vi "grabarVideoSinGuardar.vi"(0 "VideoMode":u32=20, 3 "Quality":u32=500, 5 "Stop (F)":bool, 7 "error in":errorcluster, 8 "Image Logging Path":string="C:\\Users\\TGM1603\\Documents\\Videos", 9 "Frame Rate":u32=30) -> (20 "Image Out":T1(plugin-control), 26 "Stopped":bool, 27 "error out":errorcluster)   [LabVIEW 2024]
doc: "Creates, and edits acquisitions using the NI Vision Acquisition Express VI.\n\nThe NI Vision Acquisition Wizard is launched by placing the Express VI on the block diagram. Select an acquisition source and configure an acquisition using NI-IMAQ, NI-IMAQdx, or simulate an acquisition by reading an AVI or image files from a folder. After an acquisition is configured, select controls and indicators to be able to programmatically set in LabVIEW. Double-click the Vision Acquisition Express VI to edit the acquisition.\n\nNote: Any images created by the Express VI need to be disposed after use. Use the IMAQ Dispose.vi to cleanup the images output by the Express VI when they are no longer needed."
uses:
  <vilib>/vision/driver/Vision Acquisition Express Utility VIs.llb/Vision Acquisition Path Convert (String).vi
  <vilib>/vision/driver/NI_Vision_Acquisition_Software.lvlib
  <resource>/objmgr/imaqdx.rc
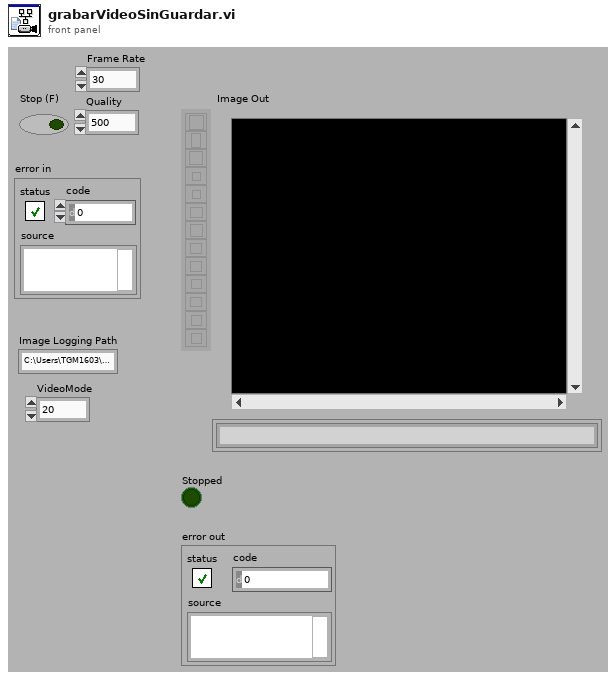
[diagram p1: front panel]
types:
  T1 = typedef "IMAQ Image.ctl" = refnum<image>
  T2 = typedef "IMAQdx.ctl" = refnum<k21>
  T3 = cluster{"File Type":string, "Quality":u32, "Compress":bool, "Lossless":bool, "Ratio":sgl, "Codec":string, "Frame Rate":u32, "Limit Frames":bool, "Max Frames":u32}
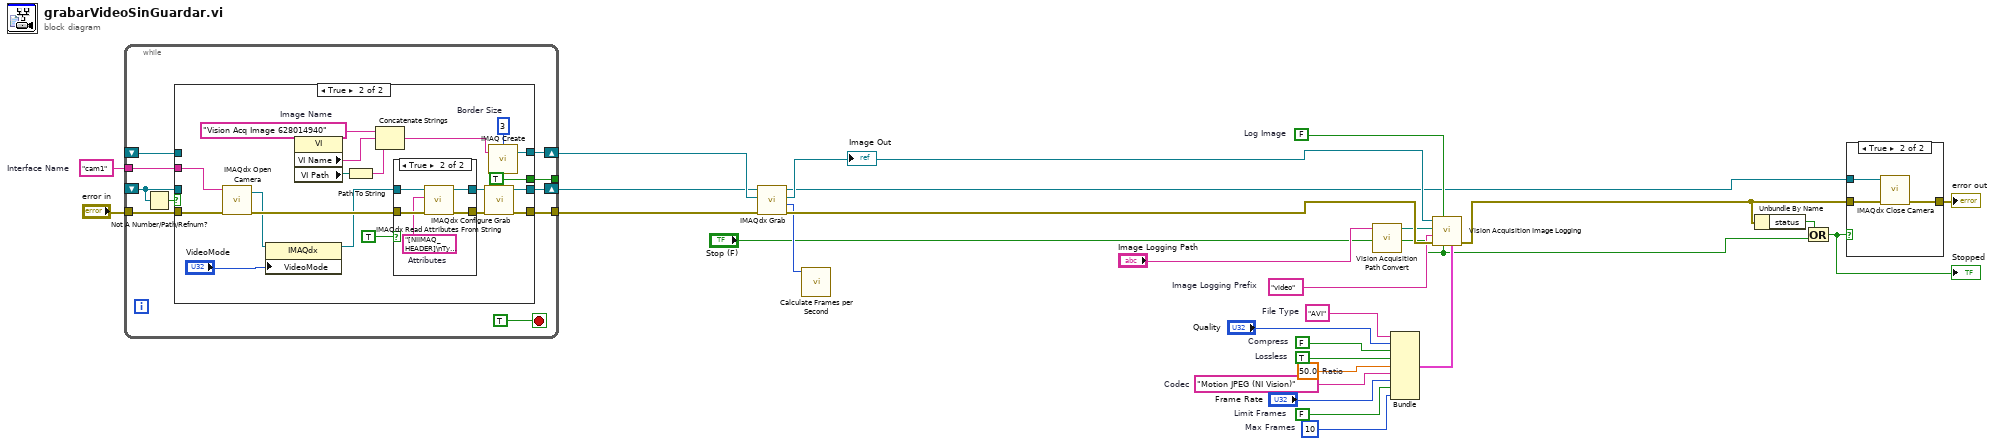
[diagram p0: block diagram]
diagram:
  w9 = FALSE  # Log Image
  w20 = "video"  # Image Logging Prefix
  w15 = sgl 50.0  # Ratio
  w16 = TRUE  # Lossless
  w17 = FALSE  # Compress
  w14 = "Motion JPEG (NI Vision)"  # Codec
  w11 = u32 10  # Max Frames
  w12 = FALSE  # Limit Frames
  w19 = "AVI"  # File Type
  w26 = "cam1"  # Interface Name
  n1 = while "While Loop_template0" {
    shift-right: [w38] -> w24
    shift-left: _ -> [w31]
    tunnel: [w37] -> w27
    tunnel: "error in" -> [w36]
    shift-right: [w34] -> w25
    shift-left: _ -> [w33]
    tunnel: w26 -> [w32]
    tunnel: [w29] -> _
    stop <- TRUE ("_template0") stop-if-true
    n2 = Not A Number/Path/Refnum?(number/path/refnum=w31) -> (NaN/Path/Refnum?=w30:bool)
    n3 = case "Case Structure_template0" shown="True" w30 {
      tunnel: [w41 w59] -> w38
      tunnel: w31 -> [w41 _]
      tunnel: [w40 w58] -> w37
      tunnel: w36 -> [w40 w60]
      tunnel: [w39 w57] -> w34
      tunnel: w33 -> [w39 _]
      tunnel: w32 -> [_ w48]
      tunnel: [_ TRUE] -> w29
      frame False {
      }
      frame True {
        w45 = 3  # Border Size
        w52 = "Vision Acq Image 628014940"  # Image Name
        n4 = call <vilib>:"IMAQdx Open Camera.vi"("error in"=w60, "Session In"=w48) -> ("error out"=w51:errorcluster, "Session Out"=w43:T2)  [unwired: 1 in, 7 out]
        n5 = property class="IMAQdx"(reference=w43, "VideoMode"="VideoMode") -> (reference out=w42:T2)  [unwired: 1 in, 1 out]
        n6 = property class="VI"() -> ("VI Name"=w55:string, "VI Path"=w56:path)  [unwired: 2 in, 2 out]
        n7 = Path To String(path=w56) -> (string=w54:string)
        n8 = Concatenate Strings(w52, w55, w54) -> (w53:string)
        n9 = case shown="True" TRUE ("Init Attributes") {
          tunnel: w42 -> [w62 w67]
          tunnel: w51 -> [w61 w66]
          tunnel: [w62 w64] -> w50
          tunnel: [w61 w63] -> w49
          frame False {
          }
          frame True {
            w65 = "[NIIMAQ_HEADER]\nType = 2\nVersion = 8\n\n[CAMERA_DATA]\nAcquisitionAttributes::Bayer::Algorithm = \"Bilinear\"\nAcquisitionAttributes::Bayer::GainB = \"1\"\nAcquisitionAttributes::Bayer::GainG = \"1\"\nAcquisitionAttributes::Bayer::GainR = \"1\"\nAcquisitionAttributes::Bayer::Pattern = \"Use hardware value\"\nAcquisitionAttributes::BitsPerPixel = \"Use hardware value\"\nAcquisitionAttributes::IgnoreFirstFrame = \"false\"\nAcquisitionAttributes::ImageDecoderCopyMode = \"Auto\"\nAcquisitionAttributes::OutputImageType = \"Auto\"\nAcquisitionAttributes::OverwriteMode = \"Get Newest\"\nAcquisitionAttributes::PixelSignedness = \"Use hardware value\"\nAcquisitionAttributes::ReceiveTimestampMode = \"None\"\nAcquisitionAttributes::ShiftPixelBits = \"false\"\nAcquisitionAttributes::SwapPixelBytes = \"false\"\nAcquisitionAttributes::Timeout = \"5000\"\nAcquisitionAttributes::VerticalMirror = \"false\"\nAcquisitionAttributes::VideoMode = \"640x360 MJPG 30.00fps\"\nCameraAttributes::BacklightCompensation::Mode = \"Manual\"\nCameraAttributes::BacklightCompensation::Value = \"false\"\nCameraAttributes::Brightness::Mode = \"Manual\"\nCameraAttributes::Brightness::Value = \"128\"\nCameraAttributes::Contrast::Mode = \"Manual\"\nCameraAttributes::Contrast::Value = \"1.28\"\nCameraAttributes::Exposure::Mode = \"Auto\"\nCameraAttributes::Focus::Mode = \"Auto\"\nCameraAttributes::Gain::Mode = \"Manual\"\nCameraAttributes::Gain::Value = \"0\"\nCameraAttributes::Pan::Mode = \"Manual\"\nCameraAttributes::Pan::Value = \"0\"\nCameraAttributes::Saturation::Mode = \"Manual\"\nCameraAttributes::Saturation::Value = \"64\"\nCameraAttributes::Sharpness::Mode = \"Manual\"\nCameraAttributes::Sharpness::Value = \"4\"\nCameraAttributes::Tilt::Mode = \"Manual\"\nCameraAttributes::Tilt::Value = \"0\"\nCameraAttributes::WhiteBalance::Mode = \"Auto\"\nCameraAttributes::Zoom::Mode = \"Manual\"\nCameraAttributes::Zoom::Value = \"100\"\n"  # Attributes
            n10 = call <vilib>:"IMAQdx Read Attributes From String.vi"("error in"=w66, "Attributes String In"=w65, "Session In"=w67) -> ("error out"=w63:errorcluster, "Session Out"=w64:T2)  [unwired: 7 out]
          }
        }
        n11 = call <vilib>:"IMAQdx Configure Grab.vi"("error in"=w49, "Session In"=w50) -> ("error out"=w58:errorcluster, "Session Out"=w59:T2)  [unwired: 1 in, 7 out]
        n12 = call "IMAQ Create"("Border Size"=w45, "Image Name"=w53) -> ("New Image"=w57:T1)  [unwired: 2 in, 2 out]
      }
    }
  }
  n13 = call <vilib>:"IMAQdx Grab.vi"("error in"=w27, "Image In"=w25, "Session In"=w24) -> ("error out"=w23:errorcluster, "Buffer Number Out"=w22:u32, "Image Out"=w21:T1, "Session Out"=w5:T2)  [unwired: 1 in, 4 out]
  "Image Out" <- w21
  n14 = call <vilib>:"Calculate Frames per Second.vi"("Buffer Number"=w22) -> ()  [unwired: 2 in, 9 out]
  n15 = call-poly <vilib>:"Vision Acquisition Path Convert.vi"("Path In"="Image Logging Path") -> ("Path Out"=w7:path)  [unwired: 10 in]
  n16 = Bundle("File Type"=w19, "Quality"="Quality", "Compress"=w17, "Lossless"=w16, "Ratio"=w15, "Codec"=w14, "Frame Rate"="Frame Rate", "Limit Frames"=w12, "Max Frames"=w11) -> (w8:T3)  [unwired: 1 out]
  n17 = call <vilib>:"Vision Acquisition Image Logging.vi"("File Settings"=w8, "Close"="Stop (F)", "Log Image"=w9, "error in (no error)"=w23, "Image Logging Prefix"=w20, "Image Logging Path"=w7, "Image In"=w21) -> ("error out"=w10:errorcluster)  [unwired: 4 out]
  n18 = Unbundle By Name(w10) -> ("status"=w1:bool)
  n19 = Or(x=w1, y="Stop (F)") -> (x .or. y?=w2:bool)
  "Stopped" <- w2
  n20 = case "Case Structure_template1" shown="True" w2 {
    tunnel: [w68 w70] -> w4
    tunnel: w10 -> [w68 w71]
    tunnel: w5 -> [_ w69]
    frame False {
    }
    frame True {
      n21 = call <vilib>:"IMAQdx Close Camera.vi"("error in"=w71, "Session In"=w69) -> ("error out"=w70:errorcluster)  [unwired: 9 out]
    }
  }
  "error out" <- w4
